vi "Map Parameter Values.vi"(11 "Actual Values Array In":dbl[](array[numeric])) -> (2 "Parameter Values":map{string, dbl}(c390))   [LabVIEW 2025, in "phlair-busch-can-bus.lvlib"]
uses:
  phlair-busch-can-bus.lvlib
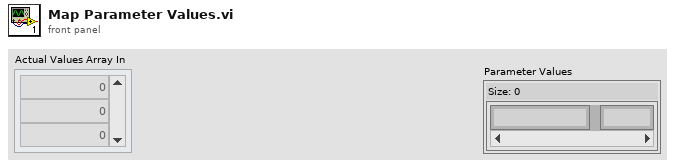
[diagram p1: front panel]
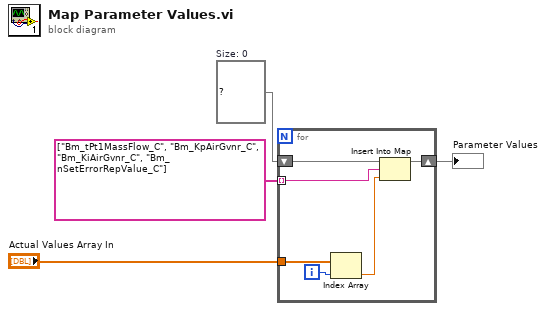
[diagram p0: block diagram]
diagram:
  w3 = map{string, dbl} {}  # Size: 0
  n1 = for {
    tunnel: string[] ["Bm_tPt1MassFlow_C", "Bm_KpAirGvnr_C", "Bm_KiAirGvnr_C", "Bm_nSetErrorRepValue_C"] -> [w10] mode=indexing
    tunnel: "Actual Values Array In" -> [w9]
    shift-right: [w6] -> w2
    shift-left: w3 -> [w5]
    i -> [w8]
    n2 = Index Array(array=w9, index=w8) -> (element=w7:dbl)
    n3 = Insert Into Map(map in=w5, key=w10, value=w7) -> (map out=w6:map{string, dbl})  [unwired: 2 out]
  }
  "Parameter Values" <- w2
